vi "Process.vi"(8 "error in":errorcluster, 11 "Plugin in":refnum<class "DateTimeChannel.lvclass">) -> (0 "error out":errorcluster, 3 "Plugin out":refnum<class "DateTimeChannel.lvclass">)   [LabVIEW 2023, in "DateTimeChannel.lvlib" / "DateTimeChannel.lvclass"]
uses:
  DateTimeChannel.lvclass
  C:/Program Files/National Instruments/LabVIEW 2023/vi.lib/FlexLogger/SDK/PluginSDK.lvlibp/PEFClasses/SDK/Plugin/Plugin.lvclass
  DateTimeChannel.lvclass/DateTimeChannel.ctl
  <vilib>/FlexLogger/SDK/PluginSDK.lvlibp/PEFClasses/SDK/Plugin/DataHelpers/Write 1D STR (NChan 1 Sample).vi
  <vilib>/FlexLogger/SDK/PluginSDK.lvlibp/PEFClasses/SDK/Plugin/Plugin.lvclass
  C:/Program Files/National Instruments/LabVIEW 2023/vi.lib/FlexLogger/SDK/PluginSDK.lvlibp/PEFClasses/SDK/Processing Element/Processing Element.lvclass
  C:/Users/bbuchana/Documents/LabVIEW Projects/FlexLogger IO Plug-ins/DateTimeChannel/DateTimeChannel.lvclass
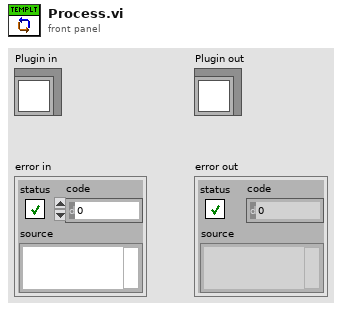
[diagram p1: front panel]
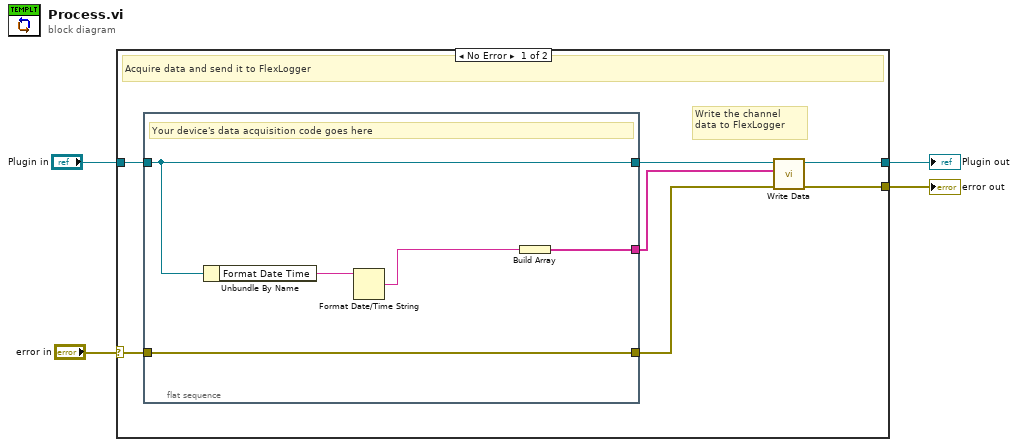
[diagram p0: block diagram]
diagram:
  n1 = case shown="No Error" "error in" {
    selector: "error in" -> [w10 w17]
    tunnel: [w6 w18] -> w4
    tunnel: "Plugin in" -> [w11 w18]
    tunnel: [w7 w17] -> w1
    frame No Error {
      # "Write the channel data to FlexLogger"
      # "Acquire data and send it to FlexLogger"
      n2 = flat-sequence {
        tunnel: [w12] -> w5
        tunnel: w11 -> [w15]
        tunnel: [w15] -> w9
        tunnel: w10 -> [w16]
        tunnel: [w16] -> w8
        frame #0 {
          # "Your device's data acquisition code goes here"
          n3 = Unbundle By Name(w15) -> ("Format Date Time"=w14:string)
          n4 = Format Date/Time String(time format string (%c)=w14) -> (date/time string=w13:string)  [unwired: 2 in]
          n5 = Build Array(w13) -> (w12:string[])
        }
      }
      n6 = call-poly <vilib>:"Write Data.vi"("error in (no error)"=w8, "Data"=w5, "Plugin in"=w9) -> ("error out"=w7:errorcluster, "Plugin out"=w6:refnum<class "DateTimeChannel.lvclass">)  [unwired: 7 in]
    }
    frame Error {
    }
  }
  "error out" <- w1
  "Plugin out" <- w4
